vi "ini_save.vi"(8 "error in":errorcluster, 11 "items to store":string) -> (0 "error out":errorcluster)   [LabVIEW 2013]
uses:
  <vilib>/Utility/config.llb/NI_LVConfig.lvlib
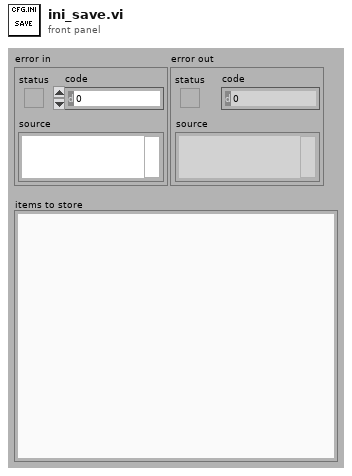
[diagram p1: front panel]
types:
  T1 = typedef "NI_LVConfig.lvlib/Config Data RefNum.ctl" = refnum<k1>
  T2 = typedef "ini_parse_row.ctl" = cluster{"ini section":string, "ini key":string, "ini default":string, "control ref":refnum<vi>, "uid":i32, "vi ref":refnum<vi>}
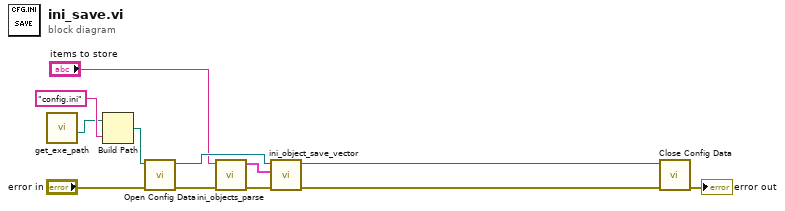
[diagram p0: block diagram]
diagram:
  n1 = call "get_exe_path.vi"() -> ("directory path"=w1:path)  [unwired: 3 out]
  n2 = Build Path(base path=w1, name or relative path="config.ini") -> (appended path=w9:path)
  n3 = call <vilib>:"Open Config Data.vi"("error in (no error)"="error in", "configuration file path"=w9) -> ("error out"=w8:errorcluster, "refnum"=w5:T1)  [unwired: 7 in, 1 out]
  n4 = call "ini_objects_parse.vi"("error in"=w8, "items command"="items to store") -> ("error out"=w7:errorcluster, "ini items"=w6:T2[])  [unwired: 8 in]
  n5 = call "ini_object_save_vector.vi"("error in"=w7, "objects to save"=w6, "refnum in"=w5) -> ("error out"=w3:errorcluster, "refnum out"=w2:T1)  [unwired: 7 in]
  n6 = call <vilib>:"Close Config Data.vi"("error in (no error)"=w3, "refnum"=w2) -> ("error out"=→"error out":errorcluster)  [unwired: 8 in, 1 out]
